vi "Apply Feedback.vi"(0 "GEA2 Reference In":refnum<k24>, 1 "Expected Modeshift Mode":string, 2 "Timeout (s)":dbl, 5 "Standalone?":bool, 7 "GEA Inputs":T1 {"Destination" format="%.0x"; "Source" format="%.0x"}, 11 "Error In":errorcluster) -> (4 "GEA2 Reference Out":refnum<k24>, 15 "Error Out":errorcluster)   [LabVIEW 2016, in "TLMB.lvlib"]
uses:
  Projects/TLMB.lvlib
  Q:/Common/DLLs/GEA3/GeaCommunication.dll
  Common/DLLs/GEA3/GeaCommunication.dll
  Common/LabVIEW GEA2 Toolkit/LabVIEW_GEA2_Toolkit.lvlibp/type defs/Source_Destination.ctl
  Common/LabVIEW GEA2 Toolkit/LabVIEW_GEA2_Toolkit.lvlibp/type defs/ERD Read Data In.ctl
  Common/LabVIEW GEA2 Toolkit/LabVIEW_GEA2_Toolkit.lvlibp/type defs/Data Type.ctl
  <vilib>/DAQmx/read.llb/DAQmx Read (Digital Bool 1Line 1Point).vi
  <vilib>/DAQmx/write.llb/DAQmx Write (Digital Bool 1Line 1Point).vi
  <vilib>/DAQmx/create/channels.llb/DAQmx Create Channel (DI-Digital Input).vi
  <vilib>/DAQmx/create/channels.llb/DAQmx Create Channel (DO-Digital Output).vi
  <vilib>/DAQmx/miscellaneous.llb/DAQmx Fill In Error Info.vi
  Common/LabVIEW GEA2 Toolkit/LabVIEW_GEA2_Toolkit.lvlibp
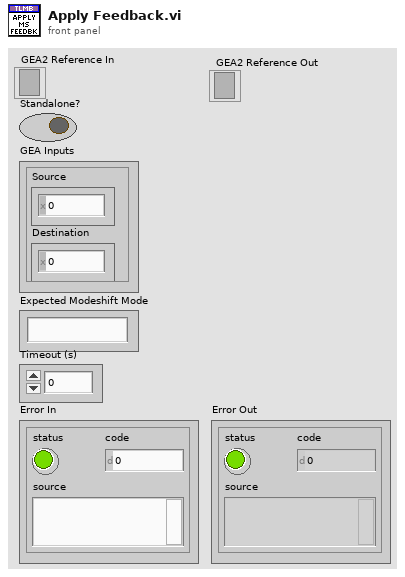
[diagram p1: front panel]
types:
  T1 = typedef "LabVIEW_GEA2_Toolkit.lvlibp/Source_Destination.ctl" = cluster{"Source":u8, "Destination":u8}
  T2 = typedef "LabVIEW_GEA2_Toolkit.lvlibp/ERD Read Data In.ctl" = cluster{"ERD Number":u16, "Data Type":T3}
  T3 = typedef "LabVIEW_GEA2_Toolkit.lvlibp/Data Type.ctl" = enum16{"string", "boolean", "uint8_t", "uint16_t", "uint32_t", "uint64_t", "int8_t", "int16_t", "int32_t", "int64_t"}
  T4 = typedef "LabVIEW_GEA2_Toolkit.lvlibp/ERD Read Data Out.ctl" = cluster{"ERD Number":u16, "Data":string}
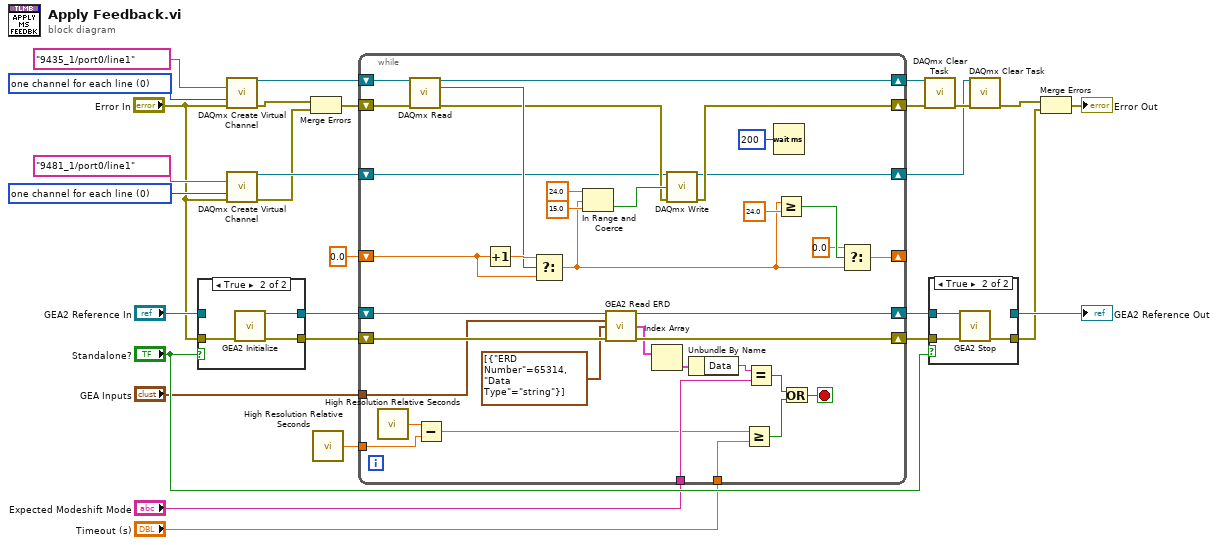
[diagram p0: block diagram]
diagram:
  w23 = 0 items=["one channel for each line", "one channel for all lines"] ("line grouping")
  w27 = 0 items=["one channel for each line", "one channel for all lines"] ("line grouping")
  n1 = case shown="True" "Standalone?" {
    tunnel: [w30 w34] -> w17
    tunnel: "Error In" -> [w31 w33]
    tunnel: [w31 w32] -> w12
    tunnel: "GEA2 Reference In" -> [w30 _]
    frame False {
    }
    frame True {
      n2 = call "GEA2 Initialize.vi"("error in"=w33) -> ("GEA2 Reference Out"=w34:refnum<k24>, "error out"=w32:errorcluster)  [unwired: 12 in, 1 out]
    }
  }
  n3 = call-poly <vilib>:"DAQmx Create Virtual Channel.vi"("lines"=tag "9435_1/port0/line1", "line grouping"=w27, "error in"="Error In") -> ("task out"=w29:refnum<k21>, "error out"=w14:errorcluster)  [unwired: 11 in]
  n4 = call-poly <vilib>:"DAQmx Create Virtual Channel.vi"("lines"=tag "9481_1/port0/line1", "line grouping"=w23, "error in"="Error In") -> ("task out"=w25:refnum<k21>, "error out"=w11:errorcluster)  [unwired: 11 in]
  n5 = Merge Errors(w14, w11) -> (w13:errorcluster)
  n6 = call <vilib>:"High Resolution Relative Seconds.vi"() -> ("relative seconds"=w6:dbl)
  n7 = while {
    shift-right: [w54] -> _
    shift-left: 0.0 -> [w64]
    shift-right: [w60] -> w22
    shift-left: w13 -> [w69]
    shift-right: [w52] -> w20
    shift-left: w29 -> [w70]
    shift-right: [w59] -> w19
    shift-left: w25 -> [w58]
    shift-right: [w48] -> w10
    shift-left: w12 -> [w49]
    shift-right: [w50] -> w18
    shift-left: w17 -> [w51]
    tunnel: "GEA Inputs" -> [w44]
    tunnel: "Expected Modeshift Mode" -> [w42]
    tunnel: w6 -> [w36]
    tunnel: "Timeout (s)" -> [w35]
    stop <- w40 stop-if-true
    n8 = call <vilib>:"High Resolution Relative Seconds.vi"() -> ("relative seconds"=w39:dbl)
    n9 = call-poly <vilib>:"DAQmx Read.vi"("task/channels in"=w70, "error in"=w69) -> ("task out"=w52:refnum<k21>, "data"=w63:bool, "error out"=w61:errorcluster)  [unwired: 11 in]
    n10 = Subtract(x=w39, y=w36) -> (x-y=w37:dbl)
    n11 = Increment(x=w64) -> (x+1=w65:dbl)
    n12 = Select(t=w65, s=w63, f=w64) -> (s? t:f=w56:dbl)
    n13 = In Range and Coerce(upper limit=24.0, x=w56, lower limit=15.0) -> (In Range?=w62:bool)  [unwired: 1 out]
    n14 = call "GEA2 Read ERD.vi"("GEA2 Reference In"=w51, "GEA Inputs"=w44, "Read ERD List"=T2[] [{"ERD Number"=65314, "Data Type"=enum."string"}], "Error In"=w49) -> ("GEA2 Reference Out"=w50:refnum<k24>, "ERD Data Out"=w47:T4[], "Error Out"=w48:errorcluster)  [unwired: 8 in, 1 out]
    n15 = Index Array(array=w47) -> (element=w46:T4)  [unwired: 1 in]
    n16 = call-poly <vilib>:"DAQmx Write.vi"("task/channels in"=w58, "data"=w62, "error in"=w61) -> ("task out"=w59:refnum<k21>, "error out"=w60:errorcluster)  [unwired: 10 in, 1 out]
    n17 = Unbundle By Name(w46) -> ("Data"=w43:string)
    n18 = Greater Or Equal?(x=w37, y=w35) -> (x >= y?=w38:bool)
    n19 = Equal?(x=w43, y=w42) -> (x = y?=w41:bool)
    n20 = Wait (ms)(milliseconds to wait=u32 200) -> ()  [unwired: 1 out]
    n21 = Greater Or Equal?(x=w56, y=24.0) -> (x >= y?=w57:bool)
    n22 = Or(x=w41, y=w38) -> (x .or. y?=w40:bool)
    n23 = Select(t=0.0, s=w57, f=w56) -> (s? t:f=w54:dbl)
  }
  n24 = call <vilib>:"DAQmx Clear Task.vi"("task in"=w20, "error in"=w22) -> ("error out"=w21:errorcluster)  [unwired: 13 in]
  n25 = case shown="True" "Standalone?" {
    tunnel: w18 -> [w72 w75]
    tunnel: w10 -> [w71 w74]
    tunnel: [w72 _] -> w8
    tunnel: [w71 w73] -> w3
    frame False {
    }
    frame True {
      n26 = call "GEA2 Stop.vi"("GEA2 Reference In"=w75, "Error In"=w74) -> ("Error Out"=w73:errorcluster)  [unwired: 13 in]
    }
  }
  "GEA2 Reference Out" <- w8
  n27 = call <vilib>:"DAQmx Clear Task.vi"("task in"=w19, "error in"=w21) -> ("error out"=w4:errorcluster)  [unwired: 13 in]
  n28 = Merge Errors(w4, w3) -> (→"Error Out":errorcluster)
